vi "Test serial monitor-v2.vi"() -> ()   [LabVIEW 2019]
uses:
  <vilib>/Platform/TimedLoop/XDataNode/timing_clust.ctl
  <vilib>/Platform/TimedLoop/XDataNode/nitl_modes.ctl
  <vilib>/Platform/TimedLoop/XDataNode/wakeup.ctl
  <vilib>/Instr/_visa.llb/VISA Configure Serial Port (Instr).vi
  <vilib>/Utility/inputDevices.llb/joystickAcquire.vi
  <vilib>/Utility/inputDevices.llb/closeJoystick.vi
  <vilib>/platform/TimedLoop/XDataNode/XDataNode.xnode
  <vilib>/Platform/TimedLoop/XDataNode/XDNodeRunTimeDep.lvlib
panel:
  out "subarray 2":dbl[](array[numeric])
  out "read buffer 2":string
  out "spreadsheet string":string
  out "axis info 2":T1
  in  "device index 2":i32
  out "button info":T2
  in  "Stop":bool
  in  "VISA resource name":refnum<visa-resource-name>
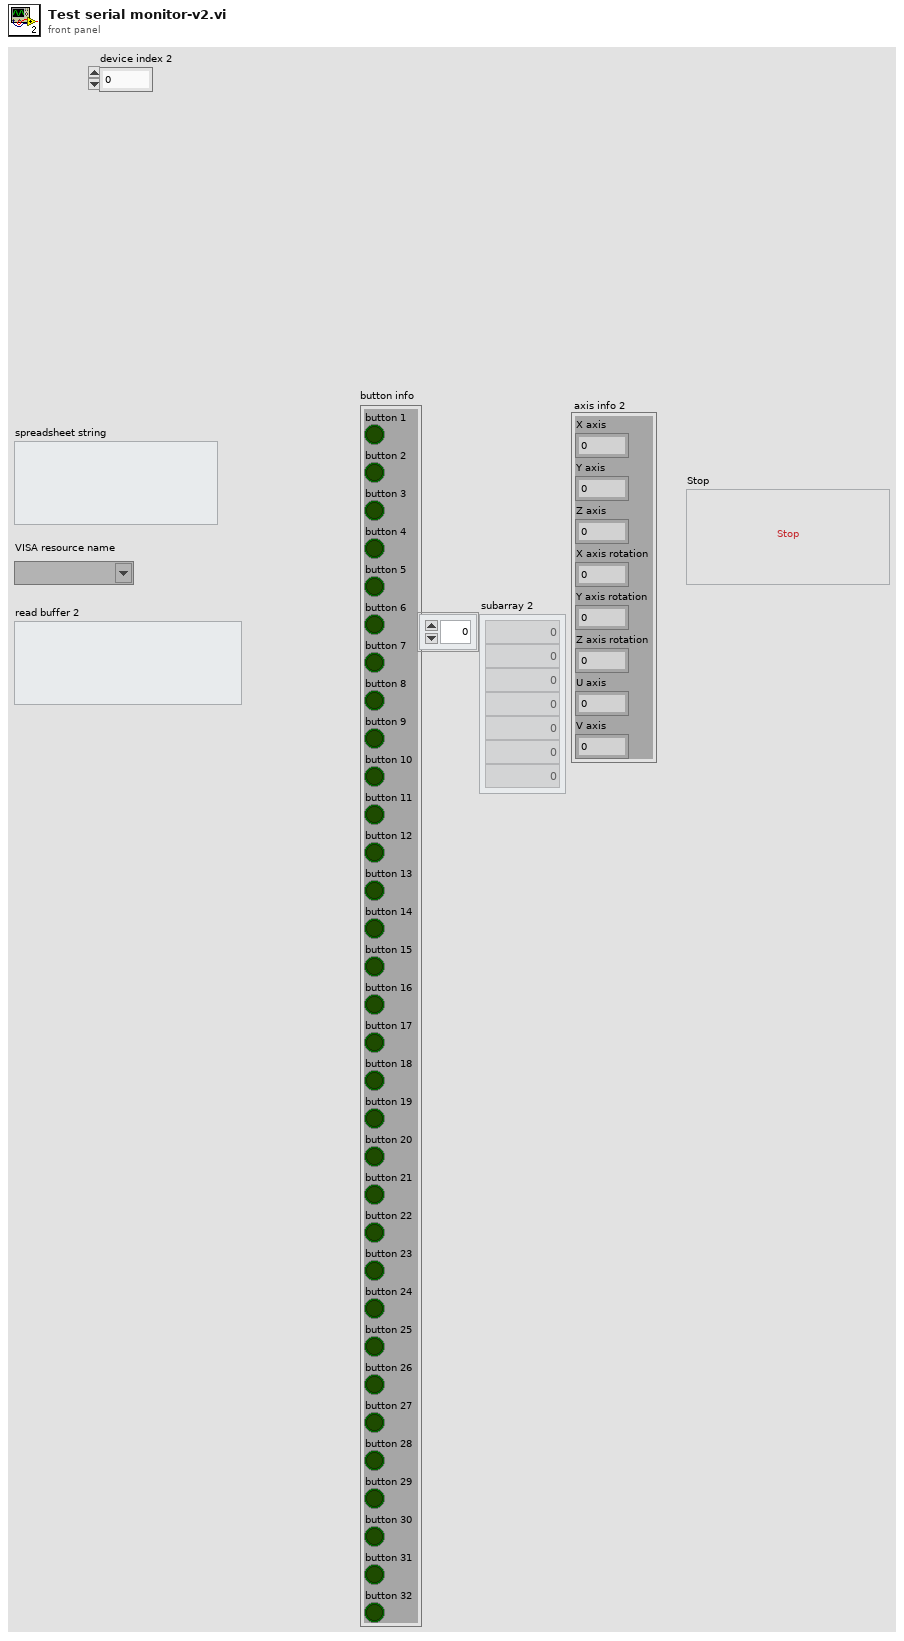
[diagram p1: front panel]
types:
  T1 = cluster{"X axis":i32, "Y axis":i32, "Z axis":i32, "X axis rotation":i32, "Y axis rotation":i32, "Z axis rotation":i32, "U axis":i32, "V axis":i32}
  T2 = cluster{"button 1":bool, "button 2":bool, "button 3":bool, "button 4":bool, "button 5":bool, "button 6":bool, "button 7":bool, "button 8":bool, "button 9":bool, "button 10":bool, "button 11":bool, "button 12":bool, "button 13":bool, "button 14":bool, "button 15":bool, "button 16":bool, "button 17":bool, "button 18":bool, "button 19":bool, "button 20":bool, "button 21":bool, "button 22":bool, "button 23":bool, "button 24":bool, "button 25":bool, "button 26":bool, "button 27":bool, "button 28":bool, "button 29":bool, "button 30":bool, "button 31":bool, "button 32":bool}
  T3 = typedef "XDNodeRunTimeDep.lvlib/timing_clust.ctl" = cluster{"Expected End [f-1]":u64, "Actual End [f-1]":u64, "Finished Late? [f-1]":bool, "Expected End [i-1]":u64, "Actual End [i-1]":u64, "Finished Late? [i-1]":bool, "Expected Start [i]":u64, "Actual Start [i]":u64, "Expected Start [f]":u64, "Actual Start [f]":u64, "Source Name":string, "Structure Name":string, "Period":i64, "Deadline":i64, "Offset":i64, "Start":i64, "Priority":i32, "Timeout":i32, "Mode":T4, "Wakeup Reason":T5, "Error":errorcluster, "Source Type":string, "Secondary Source Type":string, "Global End Time":u64, "Global Start Time":u64, "Frame Duration":u64, "Iteration Duration":u64, "Assigned CPU":i32, "I/O Scan Engine Mode":u32}
  T4 = typedef "XDNodeRunTimeDep.lvlib/nitl_modes.ctl" = enum32{"No Change", "Process missed periods, maintain original phase", "Discard missed periods, maintain original phase", "Process missed periods, ignore original phase", "Discard missed periods, ignore original phase"}
  T5 = typedef "XDNodeRunTimeDep.lvlib/wakeup.ctl" = enum32{"Normal", "Aborted", "Asynchronous wakeup", "Timing source error", "Timed loop error", "Timeout"}
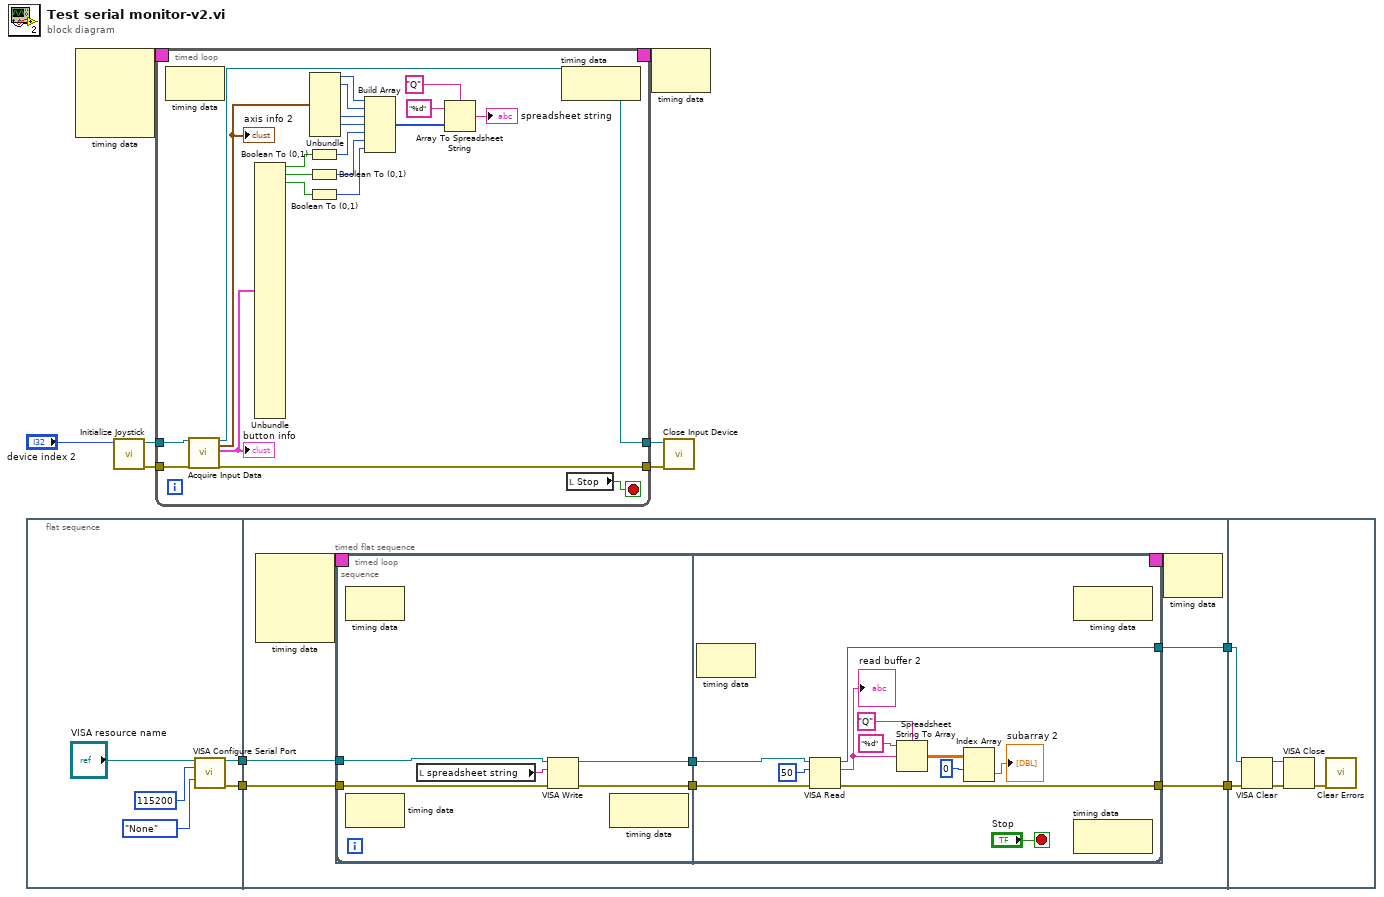
[diagram p0: block diagram]
diagram:
  n1 = flat-sequence {
    tunnel: [w13] -> w6
    tunnel: [w12] -> w5
    tunnel: w6 -> [w20]
    tunnel: w5 -> [w19]
    tunnel: [w18] -> w4
    tunnel: [w17] -> w3
    tunnel: w4 -> [w59]
    tunnel: w3 -> [w58]
    frame #0 {
      n2 = call-poly "VISA Configure Serial Port"("VISA resource name"="VISA resource name", "baud rate (9600)"=u32 115200, "parity (0:none)"=enum16{"None", "Odd", "Even", "Mark", "Space"}."None") -> ("VISA resource name out"=w13:refnum<visa-resource-name>, "error out"=w12:errorcluster)  [unwired: 11 in]
    }
    frame #1 {
      n3 = node-c288() -> (w22:T3)  [unwired: 4 in]
      n4 = timed-loop {
        tunnel: w20 -> [w26]
        tunnel: w19 -> [w25]
        timing: w22 -> [_]
        timing-out: [_] -> w21
        tunnel: [w24] -> w18
        tunnel: [w23] -> w17
        stop <- "Stop" stop-if-true
        n5 = timed-sequence {
          timing: _ -> [_]
          timing-out: _ -> [_]
          tunnel: w26 -> [w32]
          tunnel: w25 -> [w31]
          tunnel: [w28] -> w24
          tunnel: [w27] -> w23
          n6 = timed-flat-sequence {
            tunnel: w32 -> [w37]
            tunnel: w31 -> [w36]
            tunnel: [w34] -> w30
            tunnel: [w33] -> w29
            tunnel: w30 -> [w41]
            tunnel: w29 -> [w40]
            tunnel: [w43] -> w28
            tunnel: [w42] -> w27
            frame #0 {
              n7 = node-c288() -> ()  [unwired: 1 in, 1 out]
              n8 = local read "spreadsheet string"() -> (w35:string)
              n9 = VISA Write(VISA resource name=w37, write buffer=w35, error in (no error)=w36) -> (VISA resource name out=w34:refnum<visa-resource-name>, error out=w33:errorcluster)  [unwired: 1 out]
              n10 = node-c288() -> ()  [unwired: 1 in, 1 out]
            }
            frame #1 {
              n11 = node-c288() -> ()  [unwired: 1 in, 1 out]
              n12 = VISA Read(VISA resource name=w41, byte count=u32 50, error in (no error)=w40) -> (VISA resource name out=w43:refnum<visa-resource-name>, read buffer=w44:string, error out=w42:errorcluster)  [unwired: 1 out]
              "read buffer 2" <- w44
              n13 = Spreadsheet String To Array(delimiter (Tab)="Q", format string="%d", spreadsheet string=w44) -> (array=w47:dbl[][])  [unwired: 1 in]
              n14 = Index Array(array=w47, index (row)=0) -> (element=→"subarray 2":dbl[])  [unwired: 1 in]
              n15 = node-c288() -> ()  [unwired: 1 in, 1 out]
            }
          }
        }
        n16 = node-c288() -> ()  [unwired: 1 in, 1 out]
        n17 = node-c288() -> ()  [unwired: 1 in, 1 out]
      }
      n18 = node-c288(w21) -> ()  [unwired: 1 out]
    }
    frame #2 {
      n19 = VISA Clear(VISA resource name=w59, error in (no error)=w58) -> (VISA resource name out=w61:refnum<visa-resource-name>, error out=w60:errorcluster)
      n20 = VISA Close(VISA resource name=w61, error in (no error)=w60) -> (error out=w62:errorcluster)
      n21 = call <vilib>:"Clear Errors.vi"("error in (no error)"=w62) -> ()  [unwired: 5 in, 2 out]
    }
  }
  n22 = node-c288() -> (w2:T3)  [unwired: 4 in]
  n23 = call <vilib>:"Initialize Joystick.vi"("device index"="device index 2") -> ("error out"=w7:errorcluster, "device ID"=w10:refnum<k1>)  [unwired: 9 in]
  n24 = timed-loop {
    tunnel: w10 -> [w82]
    tunnel: [w81] -> w9
    tunnel: [w80] -> w8
    tunnel: w7 -> [w79]
    timing: w2 -> [_]
    timing-out: [_] -> w1
    stop <- w83 stop-if-true
    n25 = node-c288() -> ()  [unwired: 1 in, 1 out]
    n26 = call-poly <vilib>:"Acquire Input Data.vi"("device ID"=w82, "error in (no error)"=w79) -> ("device ID"=w81:refnum<k1>, "axis info"=w77:T1, "button info"=w78:T2, "error out"=w80:errorcluster)  [unwired: 13 in, 1 out]
    "button info" <- w78
    "axis info 2" <- w77
    n27 = Unbundle(w78) -> ("button 1"=w72:bool, "button 2"=w71:bool, "button 3"=w70:bool)  [unwired: 29 out]
    n28 = Boolean To (0,1)(Boolean=w72) -> (0, 1=w69:i16)
    n29 = Boolean To (0,1)(Boolean=w71) -> (0, 1=w68:i16)
    n30 = Boolean To (0,1)(Boolean=w70) -> (0, 1=w67:i16)
    n31 = Unbundle(w77) -> ("X axis"=w76:i32, "Y axis"=w75:i32, "Z axis rotation"=w74:i32, "U axis"=w73:i32)  [unwired: 4 out]
    n32 = Build Array(w76, w75, w74, w73, w69, w68, w67) -> (w64:i32[])
    n33 = Array To Spreadsheet String(delimiter (Tab)="Q", array=w64, 3:"%d" ("format string")) -> (spreadsheet string=→"spreadsheet string":string)
    n34 = node-c288() -> ()  [unwired: 1 in, 1 out]
    n35 = local read "Stop"() -> (w83:bool)
  }
  n36 = node-c288(w1) -> ()  [unwired: 1 out]
  n37 = call-poly <vilib>:"Close Input Device.vi"("error in (no error)"=w8, "device ID"=w9) -> ()  [unwired: 8 in, 1 out]
